vi "ROI corrector.vi"(10 "ROI":u8[][](array[numeric]), 11 "Spot diameter":i32) -> (3 "Corrected ROI":u8[][](array[numeric]))   [LabVIEW 2016]
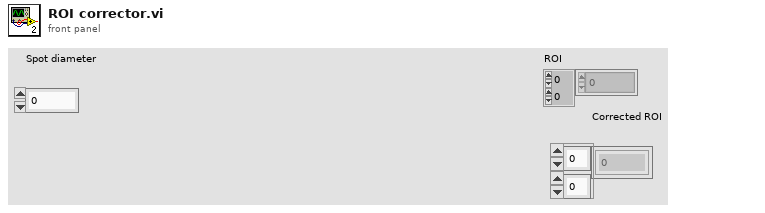
[diagram p1: front panel]
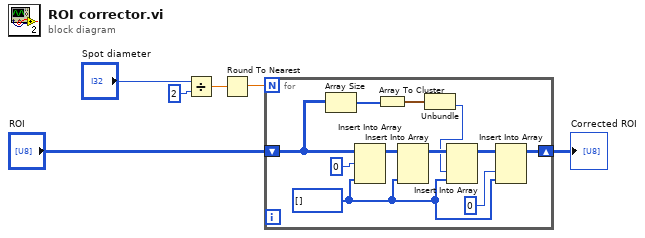
[diagram p0: block diagram]
diagram:
  n1 = Divide(x="Spot diameter", y=2) -> (x/y=w6:dbl)
  n2 = Round To Nearest(number=w6) -> (nearest integer value=w3:dbl)
  n3 = for {
    N: w3 -> [_]
    shift-right: [w12] -> w1
    shift-left: "ROI" -> [w8]
    w13 = u8[] [] ("new element/subarray")
    n4 = Array Size(array=w8) -> (size(s)=w9:i32[])
    n5 = Insert Into Array(array=w8, index (row)=0, new element=w13) -> (w16:u8[][])  [unwired: 1 in]
    n6 = Array To Cluster(array=w9) -> (cluster=w10:cluster{"[0]":i32, "[1]":i32})
    n7 = Insert Into Array(array=w16, new element=w13) -> (w15:u8[][])  [unwired: 2 in]
    n8 = Unbundle(w10) -> ("[1]"=w7:i32)  [unwired: 1 out]
    n9 = Insert Into Array(array=w15, index (col)=w7, new element=w13) -> (w14:u8[][])  [unwired: 1 in]
    n10 = Insert Into Array(array=w14, index (col)=0 ("disabled index (col)"), new element=w13) -> (w12:u8[][])  [unwired: 1 in]
  }
  "Corrected ROI" <- w1
